vi "Acquire Data Core.vi"(8 "Error In":errorcluster, 11 "LHW-DataGenerator-Actor in":refnum<class "LHW-DataGenerator-Actor.lvclass">) -> (0 "Error Out":errorcluster, 2 "LHW-DataCollection":refnum<class "LHW-DataCollection.lvclass">, 3 "LHW-DataGenerator-Actor out":refnum<class "LHW-DataGenerator-Actor.lvclass">)   [LabVIEW 2014, in "LHW-DataGenerator.lvlib" / "LHW-DataGenerator-Actor.lvclass"]
doc: "Acquire Data."
uses:
  LHW-DataGenerator-Actor.lvclass
  Classes/LHW-Data/LHW-DataCollection/LHW-DataCollection.lvclass
  Classes/LHW-Data/LHW-WfmData/LHW-WfmData.lvclass
  Classes/LHW-Data/LHW-Data/LHW-Data.lvclass/LHW-Data.ctl
  Classes/LHW-Data/LHW-WfmData/LHW-WfmData.lvclass/LHW-WfmData.ctl
  Classes/LHW-Data/LHW-DataCollection/LHW-DataCollection.lvclass/LHW-DataCollection.ctl
  <vilib>/measure/NI_MABase.lvlib
  Classes/LHW-Data/LHW-Data/LHW-Data.lvclass
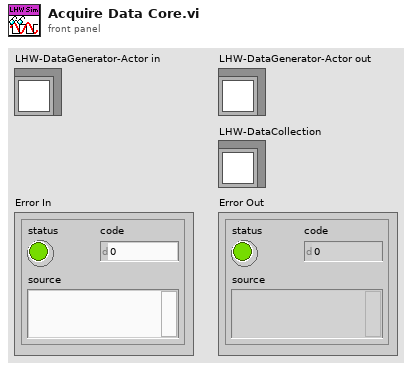
[diagram p1: front panel]
types:
  T1 = enum16{"Sine Wave", "Triangle Wave", "Square Wave", "Sawtooth Wave"}
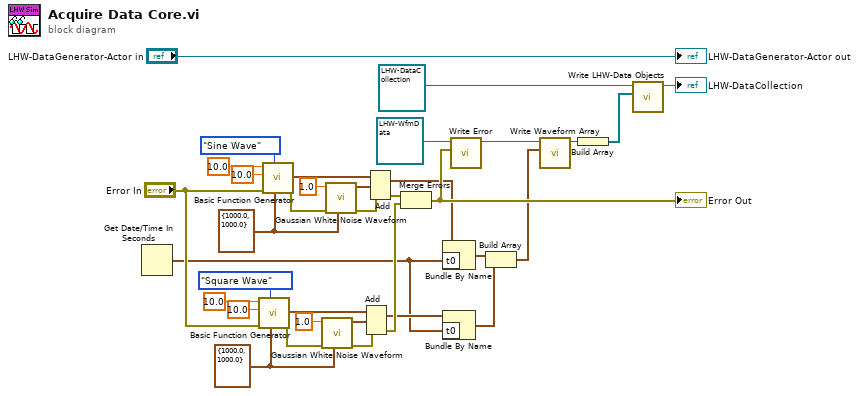
[diagram p0: block diagram]
diagram:
  w19 = cluster{"Fs":dbl, "#s":dbl} {"Fs"=1000.0, "#s"=1000.0} ("sampling info")
  w31 = cluster{"Fs":dbl, "#s":dbl} {"Fs"=1000.0, "#s"=1000.0} ("sampling info")
  n1 = Get Date/Time In Seconds() -> (seconds since 1Jan1904=w1:timestamp)
  n2 = call <vilib>:"Basic Function Generator.vi"("sampling info"=w19, "signal type"=T1."Square Wave", "error in (no error)"="Error In", "amplitude"=10.0, "frequency"=10.0) -> ("error out"=w20:errorcluster, "signal out"=w22:waveform(dbl))  [unwired: 4 in, 1 out]
  n3 = call <vilib>:"Basic Function Generator.vi"("sampling info"=w31, "signal type"=T1."Sine Wave", "error in (no error)"="Error In", "amplitude"=10.0, "frequency"=10.0) -> ("error out"=w30:errorcluster, "signal out"=w28:waveform(dbl))  [unwired: 4 in, 1 out]
  n4 = call <vilib>:"Gaussian White Noise Waveform.vi"("sampling info"=w19, "error in (no error)"=w20, "standard deviation"=1.0) -> ("error out"=w24:errorcluster, "signal out"=w23:waveform(dbl))  [unwired: 7 in]
  n5 = call <vilib>:"Gaussian White Noise Waveform.vi"("sampling info"=w31, "error in (no error)"=w30, "standard deviation"=1.0) -> ("error out"=w26:errorcluster, "signal out"=w27:waveform(dbl))  [unwired: 7 in]
  n6 = Add(1:w23, 2:w22, 4:w24) -> (0:w5:waveform(dbl), 3:w15:errorcluster)
  n7 = Add(1:w27, 2:w28, 4:w26) -> (0:w3:waveform(dbl), 3:w25:errorcluster)
  n8 = Merge Errors(w25, w15) -> (w13:errorcluster)
  "Error Out" <- w13
  n9 = Bundle By Name(cluster=w3, "t0"=w1) -> (w2:waveform(dbl))
  n10 = Bundle By Name(cluster=w5, "t0"=w1) -> (w4:waveform(dbl))
  n11 = call "Write Error.vi"("Error"=w13, "LHW-Data in"=refnum<class "LHW-WfmData.lvclass"> refnum ("LHW-Data.lvlib:LHW-WfmData.lvclass")) -> ("LHW-Data out"=w12:refnum<class "LHW-WfmData.lvclass">)  [unwired: 8 in, 1 out]
  n12 = Build Array(w2, w4) -> (w11:waveform(dbl)[])
  n13 = call "Write Waveform Array.vi"("Waveform Array"=w11, "LHW-WfmData in"=w12) -> ("LHW-WfmData out"=w8:refnum<class "LHW-WfmData.lvclass">)  [unwired: 8 in, 1 out]
  n14 = Build Array(w8) -> (w7:refnum<class "LHW-WfmData.lvclass">[])
  n15 = call "Write LHW-Data Objects.vi"("LHW-Data Objects"=w7, "LHW-DataCollection in"=refnum<class "LHW-DataCollection.lvclass"> refnum ("LHW-Data.lvlib:LHW-DataCollection.lvclass")) -> ("LHW-DataCollection out"=→"LHW-DataCollection":refnum<class "LHW-DataCollection.lvclass">)  [unwired: 8 in, 1 out]
  "LHW-DataGenerator-Actor out" <- "LHW-DataGenerator-Actor in"
